vi "New PropertyObject.vi"(8 "error in (no error)":errorcluster, 11 "Engine in":refnum<class "Engine.lvclass">) -> (0 "error out":errorcluster, 2 "PropertyObject":refnum<class "PropertyObject.lvclass">, 3 "Engine out":refnum<class "Engine.lvclass">)   [LabVIEW 2020, in "TSnax.lvlib" / "Engine.lvclass"]
uses:
  Engine.lvclass
  Engine.lvclass/Engine.ctl
  PropertyObject/PropertyObject.lvclass
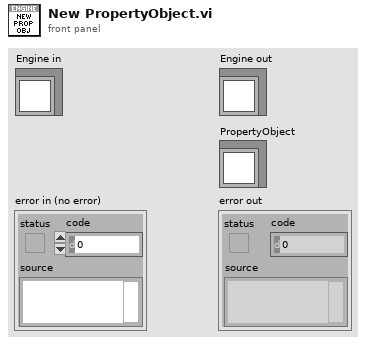
[diagram p1: front panel]
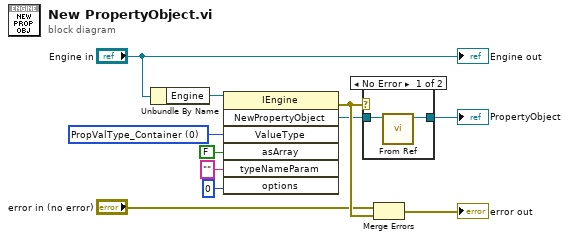
[diagram p0: block diagram]
diagram:
  w9 = 0 items=["PropValType_Container", "PropValType_String", "PropValType_Boolean", "PropValType_Number", "PropValType_NamedType", "PropValType_Reference", "PropValType_Array", "PropValType_Enum"] ("ValueType")
  n1 = Unbundle By Name("Engine in") -> ("Engine"=w4:refnum<k7>)
  n2 = invoke class="IEngine" method="NewPropertyObject"(reference=w4, "ValueType"=w9, "asArray"=FALSE, "typeNameParam"="", "options"=0) -> (error out=w11:errorcluster, "NewPropertyObject"=w3:refnum<k7>)  [unwired: 2 in, 5 out]
  n3 = case shown="No Error" w11 {
    tunnel: w3 -> [w13 _]
    tunnel: [w12 _] -> w1
    frame No Error {
      n4 = call "From Ref.vi"("PropertyObject"=w13) -> ("PropertyObject out"=w12:refnum<class "PropertyObject.lvclass">)  [unwired: 9 in, 1 out]
    }
    frame Error {
    }
  }
  "PropertyObject" <- w1
  n5 = Merge Errors("error in (no error)", w11) -> (→"error out":errorcluster)
  "Engine out" <- "Engine in"
